vi "Update Power.vi"(9 "Power (dBm)":dbl, 10 "Channel":u8=1, 11 "UI Queue in":refnum<queue>) -> (3 "UI Queue out":refnum<queue>)   [LabVIEW 2019, in "UI.lvlib"]
uses:
  UI.lvlib
  Update Message.ctl
  Update Command.ctl
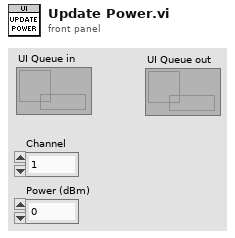
[diagram p1: front panel]
types:
  T1 = typedef "UI.lvlib/Update Command.ctl" = enum16{"Update Frequency", "Update Power", "Update Switch", "Error", "Stop"}
  T2 = typedef "UI.lvlib/Update Message.ctl" = cluster{"Update Command":T1, "Channel":u8, "Value":variant}
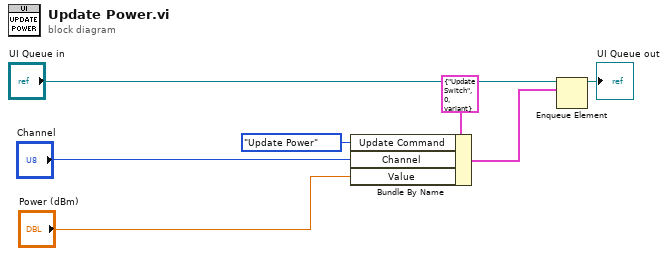
[diagram p0: block diagram]
diagram:
  n1 = Bundle By Name(cluster=T2 {"Update Command"=enum."Update Switch", "Channel"=0, "Value"=variant} ("Controller Message"), "Update Command"=Update_Command."Update Power", "Channel"="Channel", "Value"="Power (dBm)") -> (w5:T2)
  n2 = Enqueue Element(queue="UI Queue in", element=w5) -> (queue out=→"UI Queue out":refnum<queue>)  [unwired: 2 in, 2 out]
